vi "zadanie_3_drukarka.vi"() -> ()   [LabVIEW 2024]
uses:
  f2cca55d-ce66-4224-b30b-097344fa4971.vi
panel:
  out "Array":i32[](array[numeric])
  in  "String 2":string
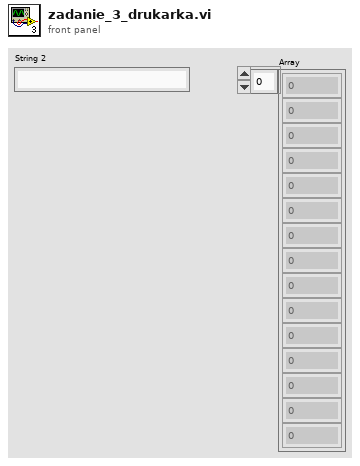
[diagram p1: front panel]
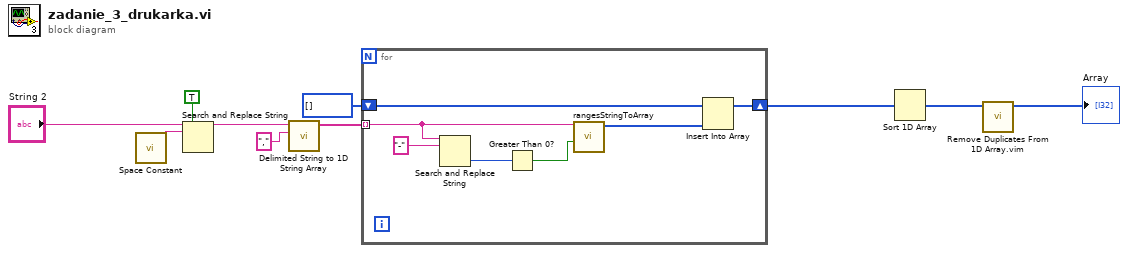
[diagram p0: block diagram]
diagram:
  n1 = call <vilib>:"Space Constant.vi"() -> ("String"=w9:string)
  n2 = Search and Replace String(replace all?=TRUE ("replace all? (F)"), input string="String 2", search string=w9) -> (result string=w7:string)  [unwired: 5 in, 3 out]
  n3 = call <vilib>:"Delimited String to 1D String Array.vi"("delimiter"=",", "delimited string"=w7) -> ("string array"=w5:string[])  [unwired: 9 in]
  n4 = for {
    tunnel: w5 -> [w14] mode=indexing
    shift-right: [w12] -> w3
    shift-left: i32[] [] -> [w11]
    n5 = Search and Replace String(input string=w14, search string="-") -> (offset past replacement=w16:i32)  [unwired: 6 in, 3 out]
    n6 = Greater Than 0?(x=w16) -> (x > 0?=w15:bool)
    n7 = call "rangesStringToArray.vi"("isThere\"-\"?"=w15, "String"=w14) -> ("Array"=w13:i32[])  [unwired: 9 in]
    n8 = Insert Into Array(array=w11, new element=w13) -> (w12:i32[])  [unwired: 1 in]
  }
  n9 = Sort 1D Array(array=w3) -> (sorted array=w2:i32[])
  n10 = call "Remove Duplicates From 1D Array.vim"("array"=w2) -> ("array with duplicates removed"=→"Array":i32[])  [unwired: 10 in]
